vi "Get Position.vi"(8 "error in (no error)":errorcluster, 11 "simulated KUKA youBot gripper motor in":refnum<class "NI_Robotics_KUKA youBot Gripper Motor_Sim.lvclass">) -> (0 "error out":errorcluster, 2 "position (m)":dbl, 3 "simulated KUKA youBot gripper motor out":refnum<class "NI_Robotics_KUKA youBot Gripper Motor_Sim.lvclass">)   [LabVIEW 2017, in "NI_Robotics_KUKA youBot Host.lvlib" / "NI_Robotics_KUKA youBot Gripper Motor_Sim.lvclass"]
uses:
  <vilib>/robotics/KUKA youBot/Motor/Gripper Motor Sim/NI_Robotics_KUKA youBot Gripper Motor_Sim.lvclass
  <vilib>/robotics/KUKA youBot/Motor/Gripper Motor Sim/NI_Robotics_KUKA youBot Gripper Motor_Sim.lvclass/NI_Robotics_KUKA youBot Gripper Motor_Sim.ctl
  <vilib>/robotics/Simulator/Interface/Simulator References/Get Joint Reference (Slider).vi
  <vilib>/robotics/Simulator/NI_Robotics_Simulator.lvlib
  <resource>/objmgr/LVODE.rc
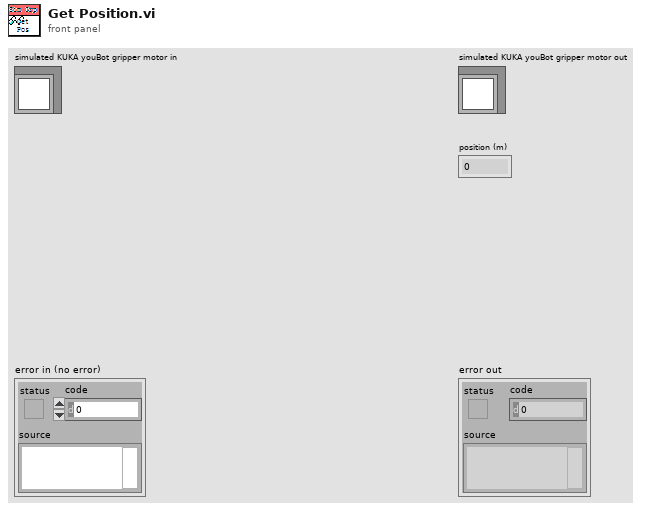
[diagram p1: front panel]
types:
  T1 = typedef "NI_Robotics_Simulator.lvlib/DeviceID.ctl" = cluster{"robot ID":string, "sensor/actuator ID":string}
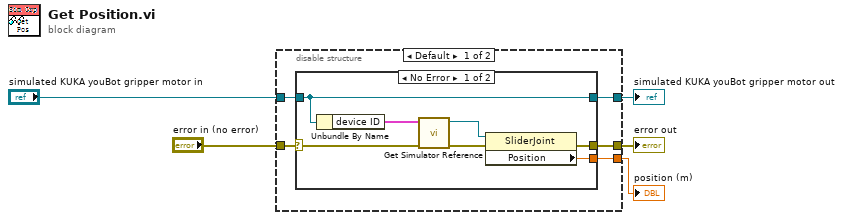
[diagram p0: block diagram]
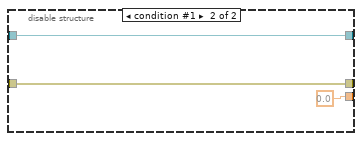
[diagram p3: hidden frame]
diagram:
  n1 = disable-structure shown="Default" {
    disable-tunnel: "simulated KUKA youBot gripper motor in" -> [w10 w22]
    disable-tunnel: "error in (no error)" -> [w9 w21]
    disable-tunnel: [w8 w22] -> w1
    disable-tunnel: [w7 0.0 ("CCW Position (rad)")] -> w3
    disable-tunnel: [w6 w21] -> w2
    frame condition #0 (active) {
      n2 = case shown="No Error" w9 {
        selector: w9 -> [w13 w19]
        tunnel: [w11 w19] -> w6
        tunnel: w10 -> [w17 w18]
        tunnel: [w17 w18] -> w8
        tunnel: [w12 _] -> w7
        frame No Error {
          n3 = Unbundle By Name(w17) -> ("device ID"=w14:T1)
          n4 = call-poly <vilib>:"Get Simulator Reference.vi"("error in (no error)"=w13, "robot joint ID"=w14) -> ("error out"=w15:errorcluster, "slider joint ref"=w16:refnum<k20>)  [unwired: 8 in]
          n5 = property class="SliderJoint"(reference=w16, error in=w15) -> (error out=w11:errorcluster, "Position"=w12:sgl)  [unwired: 1 out]
        }
        frame Error {
        }
      }
    }
    frame condition #1 {
    }
  }
  "error out" <- w2
  "simulated KUKA youBot gripper motor out" <- w1
  "position (m)" <- w3
